vi "Hysteresis-CovArrayFilter.vi"(9 "filtering":dbl format="%#_13g", 10 "Covariance Corrected":cluster{dbl, i32, i32}[][](array[cluster]), 11 "Max Hysteresis":dbl=0.2 format="%#_13g") -> (1 "Cluster filtered":cluster{dbl, i32, i32}[](array[cluster]), 2 "Covariance Values (1D)":dbl[](array[numeric]))   [LabVIEW 2016]
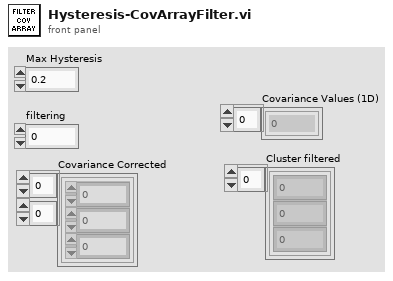
[diagram p1: front panel]
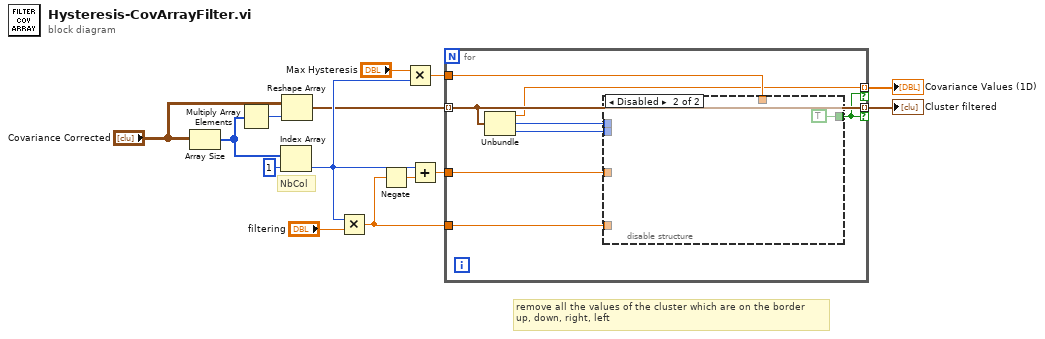
[diagram p0: block diagram]
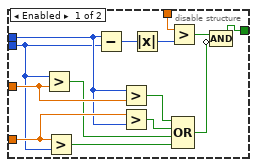
[diagram p2: hidden frame]
diagram:
  # "remove all the values of the cluster which are on the border\nup, down, right, left"
  # "NbCol"
  n1 = Array Size(array="Covariance Corrected") -> (size(s)=w3:i32[])
  n2 = Multiply Array Elements(1:w3) -> (0:w2:i32)
  n3 = Index Array(array=w3, index=1) -> (element=w13:i32)
  n4 = Reshape Array("Covariance Corrected", w2) -> (w5:cluster{dbl, i32, i32}[])
  n5 = Multiply(x=w13, y="filtering") -> (x*y=w1:dbl)
  n6 = Negate(x=w1) -> (-x=w7:dbl)
  n7 = Multiply(x="Max Hysteresis", y=w13) -> (x*y=w10:dbl)
  n8 = Add(x=w13, y=w7) -> (x+y=w8:dbl)
  n9 = for {
    tunnel: w5 -> [w20] mode=indexing
    tunnel: [w20] -> w12 mode=indexing if=w15
    tunnel: w1 -> [w22]
    tunnel: w8 -> [w21]
    tunnel: w10 -> [w17]
    tunnel: [w16] -> w11 mode=indexing if=w15
    n10 = Unbundle(w20) -> (w16:dbl, w19:i32, w18:i32)
    n11 = disable-structure shown="Disabled" {
      disable-tunnel: w22 -> [w36 _]
      disable-tunnel: w21 -> [w35 _]
      disable-tunnel: w19 -> [w29 _]
      disable-tunnel: w18 -> [w28 _]
      disable-tunnel: w17 -> [w25 _]
      disable-tunnel: [w23 TRUE] -> w15
      frame Enabled {
        n12 = Greater?(x=w28, y=w35) -> (0:w32:bool)
        n13 = Greater?(x=w36, y=w28) -> (0:w33:bool)
        n14 = Subtract(x=w29, y=w28) -> (x-y=w27:i32)
        n15 = Greater?(x=w29, y=w35) -> (0:w30:bool)
        n16 = Greater?(x=w36, y=w29) -> (0:w31:bool)
        n17 = Absolute Value(x=w27) -> (abs(x)=w26:i32)
        n18 = Greater?(x=w25, y=w26) -> (0:w24:bool)
        n19 = Compound Arithmetic op=OR(w30, w31, w32, w33) -> (w34:bool)
        n20 = Compound Arithmetic op=AND(w24, invert w34) -> (w23:bool)
      }
      frame Disabled {
      }
    }
  }
  "Cluster filtered" <- w12
  "Covariance Values (1D)" <- w11
